vi "Initialize.vi"(8 "error in (no error)":errorcluster, 11 "ELAN in":refnum<class "ELAN.lvclass">) -> (0 "error out":errorcluster, 3 "ELAN out":refnum<class "ELAN.lvclass">)   [LabVIEW 2021, in "ELAN.lvclass"]
uses:
  ELAN.lvclass
  D:/my_projects/projects/Algorithms/Labview/21/Master CR/Master CR.lvclass
  Transmission Data Unit/ELAN/ELAN Data Unit.lvclass
  Network Protocol/ELAN Master/ELAN Master.lvclass
  D:/my_projects/projects/Algorithms/Labview/21/Modbus_v121c/Network Protocol/Network Protocol.lvclass
  Transmission Data Unit/ELAN/ELAN Data Unit.lvclass/ELAN Data Unit.ctl
  Network Protocol/ELAN Master/ELAN Master.lvclass/ELAN Master.ctl
  Master CR.lvclass/Master CR.ctl
  Serial.lvclass
  ELAN.lvclass/ELAN.ctl
  Master CR.lvclass
panel:
  in  "visa resource name":refnum<visa-resource-name>="COM19"
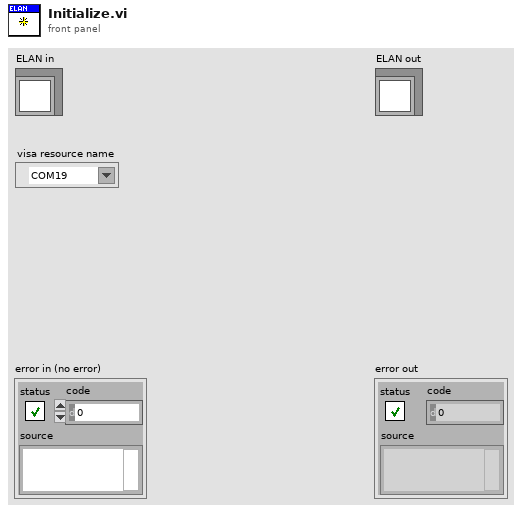
[diagram p1: front panel]
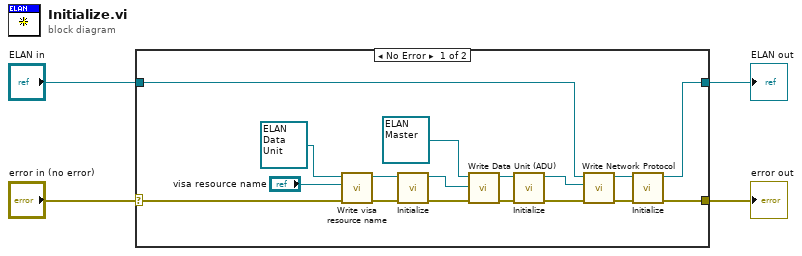
[diagram p0: block diagram]
diagram:
  n1 = case shown="No Error" "error in (no error)" {
    selector: "error in (no error)" -> [w10 w22]
    tunnel: [w20 w22] -> w1
    tunnel: [w21 w23] -> w2
    tunnel: "ELAN in" -> [w7 w23]
    frame No Error {
      n2 = call "Write visa resource name.vi"("error in (no error)"=w10, "visa resource name"="visa resource name", "ELAN Data Unit in"=refnum<class "ELAN Data Unit.lvclass"> refnum ("ASCII Data Unit")) -> ("error out"=w13:errorcluster, "ELAN Data Unit out"=w14:refnum<class "ELAN Data Unit.lvclass">)  [unwired: 7 in]
      n3 = call "Initialize.vi"("error in"=w13, "ELAN data unit (ADU) in"=w14) -> ("error out"=w19:errorcluster, "ELAN data unit (ADU) out"=w18:refnum<class "ELAN Data Unit.lvclass">)  [unwired: 8 in]
      n4 = call "Write Data Unit (ADU).vi"("error in (no error)"=w19, "ASCII Data Unit"=w18, "ELAN Master in"=refnum<class "ELAN Master.lvclass"> refnum) -> ("error out"=w16:errorcluster, "ELAN Master out"=w15:refnum<class "ELAN Master.lvclass">)  [unwired: 7 in]
      n5 = call-dynamic "Initialize.vi"("error in"=w16, "ELAN Master in"=w15) -> ("error out"=w9:errorcluster, "ELAN Master out"=w8:refnum<class "ELAN Master.lvclass">)  [unwired: 8 in]
      n6 = call "Write Network Protocol.vi"("error in (no error)"=w9, "Network Protocol"=w8, "Master CR in"=w7) -> ("error out"=w5:errorcluster, "Master CR out"=w6:refnum<class "ELAN.lvclass">)  [unwired: 7 in]
      n7 = call-parent "Initialize.vi"("error in (no error)"=w5, "Serial in"=w6) -> ("error out"=w20:errorcluster, "MB_TCP out"=w21:refnum<class "ELAN.lvclass">)  [unwired: 8 in]
    }
    frame Error {
    }
  }
  "error out" <- w1
  "ELAN out" <- w2
